vi "Channel_test_waveforms.vi"(0 "Tested channel":i32, 2 "Olfactormeter parameters":T3={"Back valve ON delays"=[0.0, 0.0, 0.0, 0.0, 0.0, 0.0, 0.0, 0.0, 0.0, 0.0, 0.0, 0.0, 0.0, 0.0, 0.0, 0.0], "Back valve OFF delays"=[0.0, 0.0, 0.0, 0.0, 0.0, 0.0, 0.0, 0.0, 0.0, 0.0, 0.0, 0.0, 0.0, 0.0, 0.0, 0.0], "Step duration (ms)"=2.0, "TTL binary step duration (ms)"=1.0, "Sampling rate (Hz)"=20000.0, "Initial delay (ms)"=250.0, "Pulse duration (ms)"=250.0} {"Initial delay (ms)" format="%#_13g"}, 3 "Odour bottles":T2(array[cluster])=[[{"Mixture components"=[{"Name"="MINERAL OIL", "CID"=0, "Volatility"=0.0}], "Name"="B1 (Bl)", "VPs"="0.0E+0", "Proportion"=[{"Numeric"=100.0}], "Selected"=FALSE, "Counter"=TRUE}, {"Mixture components"=[{"Name"="Methyl benzoate", "CID"=8103, "Volatility"=0.38}, {"Name"="Menthone", "CID"=8063, "Volatility"=0.28}], "Name"="B3 (ME2)", "VPs"="3.3E-1 ± 21%", "Proportion"=[{"Numeric"=50.0}, {"Numeric"=50.0}], "Selected"=TRUE, "Counter"=FALSE}, {"Mixture components"=[{"Name"="Decanol", "CID"=460, "Volatility"=0.00851}], "Name"="B5 (C4f)", "VPs"="8.5E-3", "Proportion"=[{"Numeric"=100.0}], "Selected"=FALSE, "Counter"=FALSE}, {"Mixture components"=[{"Name"="Acetophenone", "CID"=8174, "Volatility"=0.45}, {"Name"="Fenchone", "CID"=8635, "Volatility"=0.82}], "Name"="B7 (ME1)", "VPs"="6.4E-1 ± 41%", "Proportion"=[{"Numeric"=50.0}, {"Numeric"=50.0}], "Selected"=FALSE, "Counter"=FALSE}], [{"Mixture components"=[{"Name"="MINERAL OIL", "CID"=0, "Volatility"=0.0}], "Name"="B2 (Bl)", "VPs"="0.0E+0", "Proportion"=[{"Numeric"=100.0}], "Selected"=FALSE, "Counter"=TRUE}, {"Mixture components"=[{"Name"="Octanol", "CID"=7439, "Volatility"=0.0794}], "Name"="B4 (C4cA)", "VPs"="7.9E-2", "Proportion"=[{"Numeric"=100.0}], "Selected"=FALSE, "Counter"=FALSE}, {"Mixture components"=[{"Name"="MINERAL OIL", "CID"=0, "Volatility"=0.0}], "Name"="B6 (Bl)", "VPs"="0.0E+0", "Proportion"=[{"Numeric"=100.0}], "Selected"=FALSE, "Counter"=FALSE}, {"Mixture components"=[{"Name"="Heptanoic acid ", "CID"=957, "Volatility"=0.0107}], "Name"="B8 (C3cA)", "VPs"="1.1E-2", "Proportion"=[{"Numeric"=100.0}], "Selected"=FALSE, "Counter"=FALSE}], [{"Mixture components"=[{"Name"="MINERAL OIL", "CID"=0, "Volatility"=0.0}], "Name"="B9 (Bl)", "VPs"="0.0E+0", "Proportion"=[{"Numeric"=100.0}], "Selected"=FALSE, "Counter"=TRUE}, {"Mixture components"=[{"Name"="Geranyl acetate", "CID"=6985, "Volatility"=0.03}, {"Name"="Dimethylacetophenone", "CID"=7144, "Volatility"=0.063}], "Name"="B11 (MW1)", "VPs"="4.6E-2 ± 50%", "Proportion"=[{"Numeric"=50.0}, {"Numeric"=50.0}], "Selected"=FALSE, "Counter"=FALSE}, {"Mixture components"=[{"Name"="Geraniol", "CID"=6405, "Volatility"=0.03}, {"Name"="Phenyl butanone", "CID"=7762, "Volatility"=0.1}], "Name"="B13 (MW2)", "VPs"="6.5E-2 ± 76%", "Proportion"=[{"Numeric"=50.0}, {"Numeric"=50.0}], "Selected"=FALSE, "Counter"=FALSE}, {"Mixture components"=[{"Name"="Methylheptanoic acid", "CID"=1032, "Volatility"=0.018}], "Name"="B15 (C3f)", "VPs"="1.8E-2", "Proportion"=[{"Numeric"=100.0}], "Selected"=FALSE, "Counter"=FALSE}], [{"Mixture components"=[{"Name"="MINERAL OIL", "CID"=0, "Volatility"=0.0}], "Name"="B10 (Bl)", "VPs"="0.0E+0", "Proportion"=[{"Numeric"=100.0}], "Selected"=FALSE, "Counter"=TRUE}, {"Mixture components"=[{"Name"="Valeric acid", "CID"=8025, "Volatility"=0.196}], "Name"="B12 (C3cB)", "VPs"="2.0E-1", "Proportion"=[{"Numeric"=100.0}], "Selected"=FALSE, "Counter"=FALSE}, {"Mixture components"=[{"Name"="Nonanol", "CID"=4133, "Volatility"=0.0227}], "Name"="B14 (C4cB)", "VPs"="2.3E-2", "Proportion"=[{"Numeric"=100.0}], "Selected"=FALSE, "Counter"=FALSE}, {"Mixture components"=[{"Name"="Hydroxacetophenone", "CID"=7462, "Volatility"=0.0856}], "Name"="B16 (Ol)", "VPs"="8.6E-2", "Proportion"=[{"Numeric"=100.0}], "Selected"=FALSE, "Counter"=FALSE}]], 4 "Test type":T1(ring), 5 "Reset counters":bool) -> (7 "waveform array":digitalwaveform[](array[waveform])=[{"t0"=timestamp(0 s since 1904-01-01), "dt"=5e-05, "Y"={"transitions"=[], "data"=array5001x1[5001 elements]}, "attributes"=variant("NI_LineNames"=variant(string "Front valve 1"))}, {"t0"=timestamp(0 s since 1904-01-01), "dt"=5e-05, "Y"={"transitions"=[], "data"=array10001x1[10001 elements]}, "attributes"=variant("NI_LineNames"=variant(string "Front valve 2"))}, {"t0"=timestamp(0 s since 1904-01-01), "dt"=5e-05, "Y"={"transitions"=[], "data"=array10001x1[10001 elements]}, "attributes"=variant("NI_LineNames"=variant(string "Front valve 3"))}, {"t0"=timestamp(0 s since 1904-01-01), "dt"=5e-05, "Y"={"transitions"=[], "data"=[]}, "attributes"=variant("NI_LineNames"=variant(string "Front valve 4"))}, {"t0"=timestamp(0 s since 1904-01-01), "dt"=5e-05, "Y"={"transitions"=[], "data"=array10001x1[10001 elements]}, "attributes"=variant("NI_LineNames"=variant(string "Front valve 5"))}, {"t0"=timestamp(0 s since 1904-01-01), "dt"=5e-05, "Y"={"transitions"=[], "data"=array10001x1[10001 elements]}, "attributes"=variant("NI_LineNames"=variant(string "Front valve 6"))}, {"t0"=timestamp(0 s since 1904-01-01), "dt"=5e-05, "Y"={"transitions"=[], "data"=array10001x1[10001 elements]}, "attributes"=variant("NI_LineNames"=variant(string "Front valve 7"))}, {"t0"=timestamp(0 s since 1904-01-01), "dt"=5e-05, "Y"={"transitions"=[], "data"=array10001x1[10001 elements]}, "attributes"=variant("NI_LineNames"=variant(string "Front valve 8"))}, {"t0"=timestamp(0 s since 1904-01-01), "dt"=5e-05, "Y"={"transitions"=[], "data"=array10001x1[10001 elements]}, "attributes"=variant("NI_LineNames"=variant(string "Front valve 9"))}, {"t0"=timestamp(0 s since 1904-01-01), "dt"=5e-05, "Y"={"transitions"=[], "data"=array10001x1[10001 elements]}, "attributes"=variant("NI_LineNames"=variant(string "Front valve 10"))}, {"t0"=timestamp(0 s since 1904-01-01), "dt"=5e-05, "Y"={"transitions"=[], "data"=array10001x1[10001 elements]}, "attributes"=variant("NI_LineNames"=variant(string "Front valve 11"))}, {"t0"=timestamp(0 s since 1904-01-01), "dt"=5e-05, "Y"={"transitions"=[], "data"=array10001x1[10001 elements]}, "attributes"=variant("NI_LineNames"=variant(string "Front valve 12"))}, {"t0"=timestamp(0 s since 1904-01-01), "dt"=5e-05, "Y"={"transitions"=[], "data"=array10001x1[10001 elements]}, "attributes"=variant("NI_LineNames"=variant(string "Front valve 13"))}, {"t0"=timestamp(0 s since 1904-01-01), "dt"=5e-05, "Y"={"transitions"=[], "data"=array10001x1[10001 elements]}, "attributes"=variant("NI_LineNames"=variant(string "Front valve 14"))}, {"t0"=timestamp(0 s since 1904-01-01), "dt"=5e-05, "Y"={"transitions"=[], "data"=array10001x1[10001 elements]}, "attributes"=variant("NI_LineNames"=variant(string "Front valve 15"))}, {"t0"=timestamp(0 s since 1904-01-01), "dt"=5e-05, "Y"={"transitions"=[], "data"=array10001x1[10001 elements]}, "attributes"=variant("NI_LineNames"=variant(string "Front valve 16"))}, {"t0"=timestamp(0 s since 1904-01-01), "dt"=5e-05, "Y"={"transitions"=[], "data"=[]}, "attributes"=variant("NI_LineNames"=variant(string "Back valve 1"))}, {"t0"=timestamp(0 s since 1904-01-01), "dt"=5e-05, "Y"={"transitions"=[], "data"=[]}, "attributes"=variant("NI_LineNames"=variant(string "Back valve 2"))}, {"t0"=timestamp(0 s since 1904-01-01), "dt"=5e-05, "Y"={"transitions"=[], "data"=[]}, "attributes"=variant("NI_LineNames"=variant(string "Back valve 3"))}, {"t0"=timestamp(0 s since 1904-01-01), "dt"=5e-05, "Y"={"transitions"=[], "data"=[]}, "attributes"=variant("NI_LineNames"=variant(string "Back valve 4"))}, {"t0"=timestamp(0 s since 1904-01-01), "dt"=5e-05, "Y"={"transitions"=[], "data"=[]}, "attributes"=variant("NI_LineNames"=variant(string "Back valve 5"))}, {"t0"=timestamp(0 s since 1904-01-01), "dt"=5e-05, "Y"={"transitions"=[], "data"=[]}, "attributes"=variant("NI_LineNames"=variant(string "Back valve 6"))}, {"t0"=timestamp(0 s since 1904-01-01), "dt"=5e-05, "Y"={"transitions"=[], "data"=[]}, "attributes"=variant("NI_LineNames"=variant(string "Back valve 7"))}, {"t0"=timestamp(0 s since 1904-01-01), "dt"=5e-05, "Y"={"transitions"=[], "data"=[]}, "attributes"=variant("NI_LineNames"=variant(string "Back valve 8"))}, {"t0"=timestamp(0 s since 1904-01-01), "dt"=5e-05, "Y"={"transitions"=[], "data"=[]}, "attributes"=variant("NI_LineNames"=variant(string "Back valve 9"))}, {"t0"=timestamp(0 s since 1904-01-01), "dt"=5e-05, "Y"={"transitions"=[], "data"=[]}, "attributes"=variant("NI_LineNames"=variant(string "Back valve 10"))}, {"t0"=timestamp(0 s since 1904-01-01), "dt"=5e-05, "Y"={"transitions"=[], "data"=[]}, "attributes"=variant("NI_LineNames"=variant(string "Back valve 11"))}, {"t0"=timestamp(0 s since 1904-01-01), "dt"=5e-05, "Y"={"transitions"=[], "data"=[]}, "attributes"=variant("NI_LineNames"=variant(string "Back valve 12"))}, {"t0"=timestamp(0 s since 1904-01-01), "dt"=5e-05, "Y"={"transitions"=[], "data"=[]}, "attributes"=variant("NI_LineNames"=variant(string "Back valve 13"))}, {"t0"=timestamp(0 s since 1904-01-01), "dt"=5e-05, "Y"={"transitions"=[], "data"=[]}, "attributes"=variant("NI_LineNames"=variant(string "Back valve 14"))}, {"t0"=timestamp(0 s since 1904-01-01), "dt"=5e-05, "Y"={"transitions"=[], "data"=[]}, "attributes"=variant("NI_LineNames"=variant(string "Back valve 15"))}, {"t0"=timestamp(0 s since 1904-01-01), "dt"=5e-05, "Y"={"transitions"=[], "data"=[]}, "attributes"=variant("NI_LineNames"=variant(string "Back valve 16"))}, {"t0"=timestamp(0 s since 1904-01-01), "dt"=5e-05, "Y"={"transitions"=[], "data"=[]}, "attributes"=variant("NI_LineNames"=variant(string "Odour TTL1"))}], 10 "Test name":string)   [LabVIEW 2016]
uses:
  <vilib>/Waveform/DWDTOps.llb/DWDT Append Digital Signals.vi
panel:
  out "Digital Waveform Graph":digitalwaveform(graph)={"t0"=timestamp(0 s since 1904-01-01), "dt"=5e-05, "Y"={"transitions"=array[10001 elements], "data"=array10001x15[150015 elements]}, "attributes"=variant("NI_LineNames"=variant(string "Odour TTL1,Back valve 16,Back valve 15,Back valve 14,Back valve 13,Back valve 12,Back valve 11,Back valve 10,Back valve 9,Back valve 8,Back valve 7,Back valve 6,Back valve 5,Back valve 4,Back valve 3,Back valve 2,Back valve 1,Front valve 16,Front valve 15,Front valve 14,Front valve 13,Front valve 12,Front valve 11,Front valve 10,Front valve 9,Front valve 8,Front valve 7,Front valve 6,Front valve 5,Front valve 4,Front valve 3,Front valve 2,Front valve 1"))}
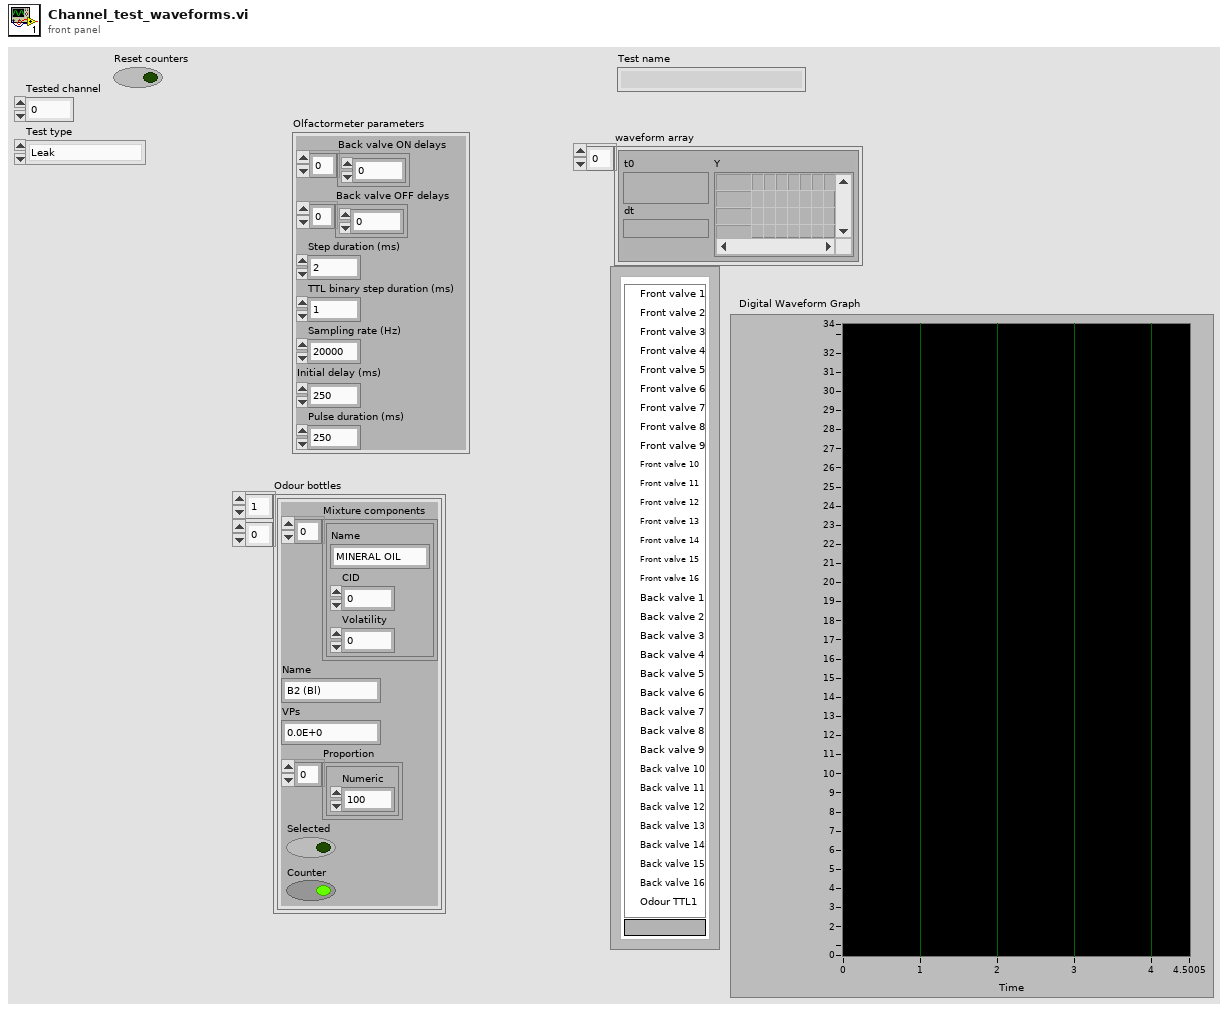
[diagram p1: front panel]
types:
  T1 = enum16{"Leak", "Flow w/o counters", "Flow w counters"}
  T2 = cluster{"Mixture components":cluster{"Name":string, "CID":i32, "Volatility":dbl}[], "Name":string, "VPs":string, "Proportion":cluster{"Numeric":dbl}[], "Selected":bool, "Counter":bool}[][]
  T3 = cluster{"Back valve ON delays":dbl[], "Back valve OFF delays":dbl[], "Step duration (ms)":dbl, "TTL binary step duration (ms)":dbl, "Sampling rate (Hz)":dbl, "Initial delay (ms)":dbl, "Pulse duration (ms)":dbl}
  T4 = cluster{"Active bottles":i32[], "Counter bottles":i32[], "All counters":i32[]}
  T5 = cluster{"Initial phase":i32, "Back-valve pre-phase ":i32, "Main phase":i32, "Back-valve post-phase":i32, "Reset":i32, "Step":i32, "Total":i32, "ON delays":i32[], "OFF delays":i32[]}
  T6 = enum16{"Inactive odour", "Active counter", "Inactive counter", "Active odour", "INVALID"}
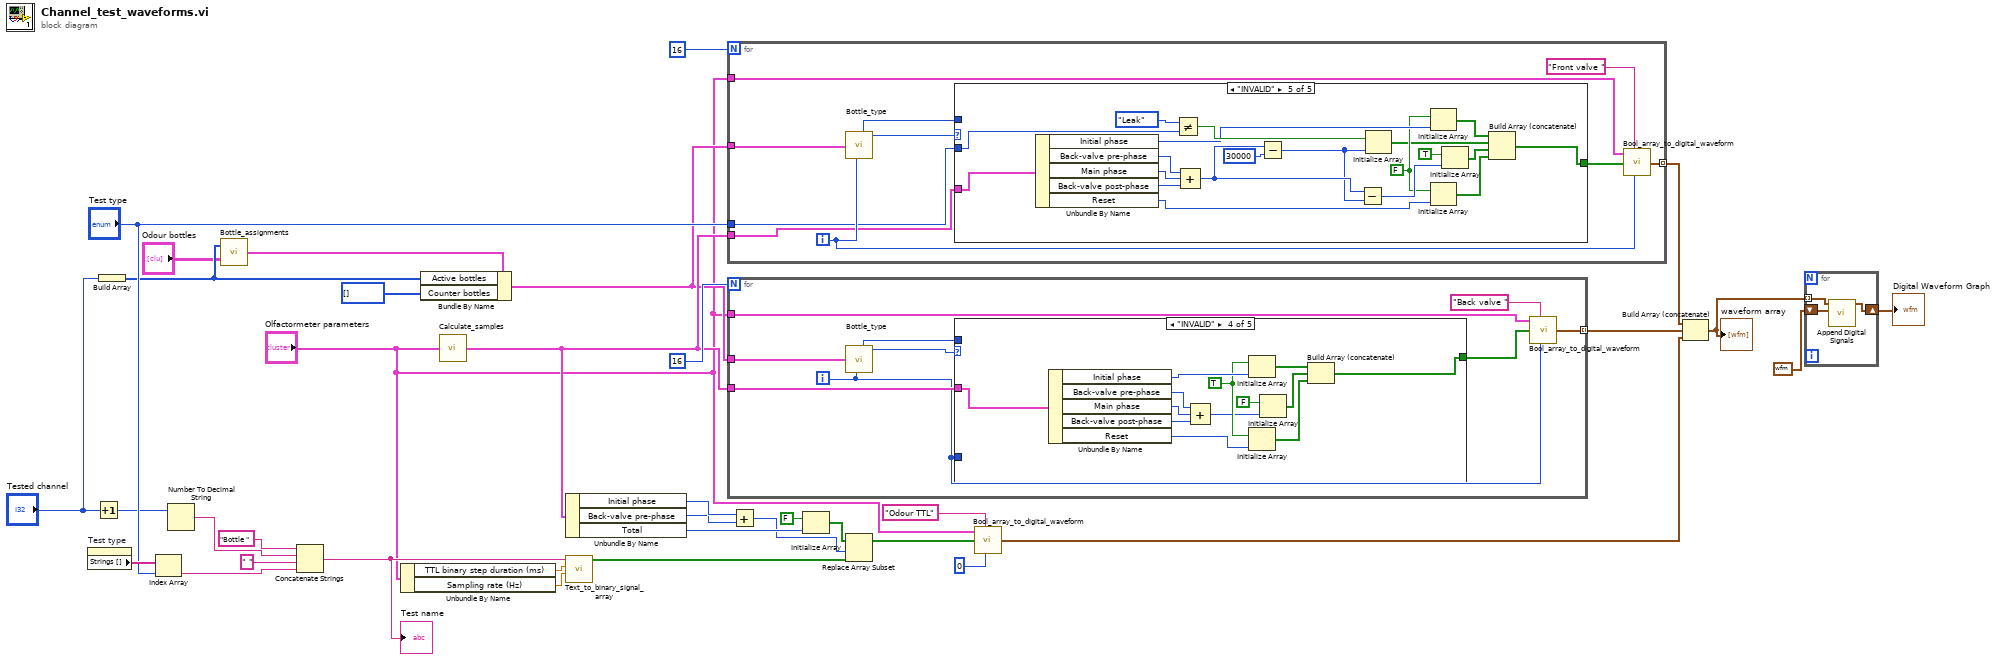
[diagram p0: block diagram]
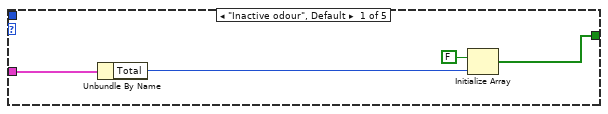
[diagram p2: hidden frame]
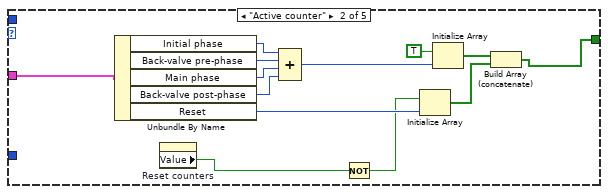
[diagram p3: hidden frame]
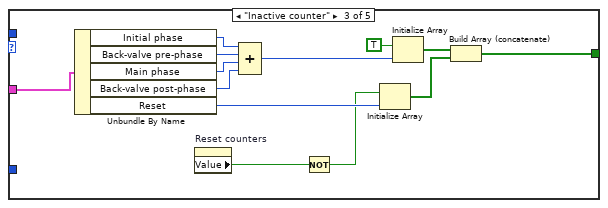
[diagram p4: hidden frame]
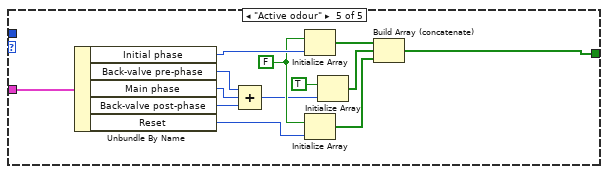
[diagram p5: hidden frame]
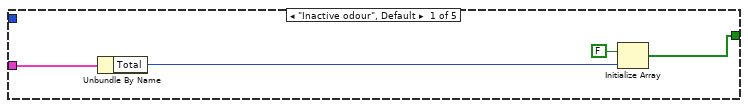
[diagram p6: hidden frame]
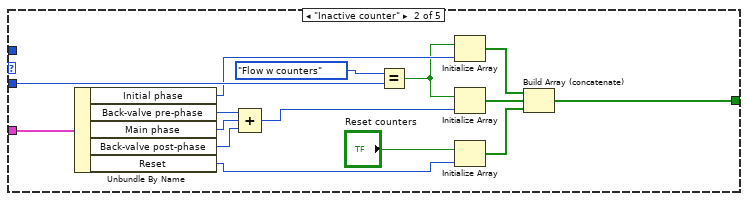
[diagram p7: hidden frame]
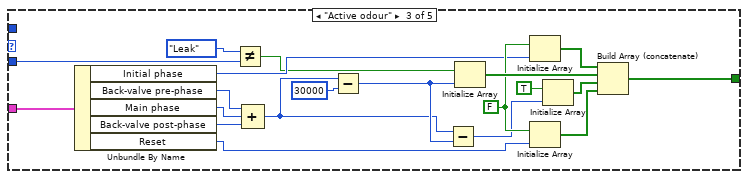
[diagram p8: hidden frame]
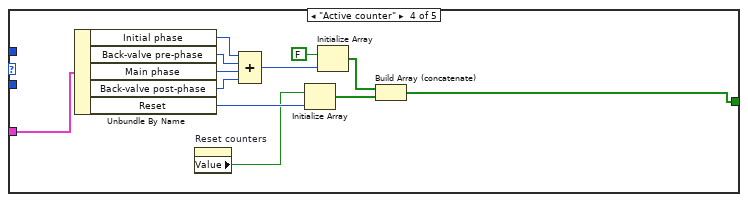
[diagram p9: hidden frame]
diagram:
  n1 = property on="Test type" class="Enum (strict)"() -> ("Strings []"=w15:string[])  [unwired: 2 in, 2 out]
  n2 = Increment(x="Tested channel") -> (x+1=w8:i32)
  n3 = Build Array("Tested channel") -> (w3:i32[])
  n4 = Index Array(array=w15, index="Test type") -> (element=w9:string)
  n5 = Number To Decimal String(number=w8) -> (decimal integer string=w11:string)  [unwired: 1 in]
  n6 = call "Bottle_assignments.vi"("Odour bottles"="Odour bottles", "Active bottles"=w3) -> ("Bottle assignments"=w1:T4)
  n7 = Concatenate Strings("Bottle " ("string"), w11, " " ("string"), w9) -> (w7:string)
  "Test name" <- w7
  n8 = Unbundle By Name("Olfactormeter parameters") -> ("TTL binary step duration (ms)"=w36:dbl, "Sampling rate (Hz)"=w33:dbl)
  n9 = Bundle By Name(cluster=w1, "Active bottles"=w3, "Counter bottles"=i32[] []) -> (w5:T4)
  n10 = call "Calculate_samples.vi"("Olfactormeter parameters"="Olfactormeter parameters") -> ("Samples"=w23:T5)  [unwired: 4 in]
  n11 = Unbundle By Name(w23) -> ("Initial phase"=w20:i32, "Back-valve pre-phase"=w19:i32, "Total"=w22:i32)
  n12 = call "Text_to_binary_signal_array.vi"("Sampling rate (Hz)"=w33, "TTL binary step duration (ms)"=w36, "Text"=w7) -> ("Signal array"=w17:bool[])  [unwired: 8 in]
  n13 = for {
    N: 16 -> [_]
    tunnel: w5 -> [w43]
    tunnel: "Olfactormeter parameters" -> [w46]
    tunnel: [w45] -> w28 mode=indexing
    tunnel: w23 -> [w40]
    tunnel: "Test type" -> [w38]
    i -> [w42]
    n14 = call "Bottle_type.vi"("Bottle assignments"=w43, "i"=w42) -> ("active bottle index"=w39:i32, "Bottle type"=w37:T6)  [unwired: 7 in]
    n15 = case shown="\"INVALID\"" w37 {
      tunnel: [w49 w56 w79 w89 w98] -> w41
      tunnel: w40 -> [w48 w57 w80 w88 w99]
      tunnel: w39 -> [_ _ _ _ _]
      tunnel: w38 -> [_ w55 w74 _ w100]
      frame "Inactive odour", Default {
        n16 = Unbundle By Name(w48) -> ("Total"=w47:i32)
        n17 = Initialize Array(FALSE, w47) -> (w49:bool[])
      }
      frame "Inactive counter" {
        n18 = Unbundle By Name(w57) -> ("Initial phase"=w52:i32, "Back-valve pre-phase"=w64:i32, "Main phase"=w63:i32, "Back-valve post-phase"=w62:i32, "Reset"=w58:i32)
        n19 = Compound Arithmetic op=ADD(w64, w63, w62) -> (w61:i32)
        n20 = Equal?(x=T1."Flow w counters", y=w55) -> (x = y?=w51:bool)
        n21 = Initialize Array(w51, w52) -> (w53:bool[])
        n22 = Initialize Array(w51, w61) -> (w60:bool[])
        n23 = Initialize Array("Reset counters", w58) -> (w59:bool[])
        n24 = Build Array (concatenate)(w53, w60, w59) -> (w56:bool[])
      }
      frame "Active odour" {
        w78 = FALSE
        n25 = Unbundle By Name(w80) -> ("Initial phase"=w77:i32, "Back-valve pre-phase"=w81:i32, "Main phase"=w82:i32, "Back-valve post-phase"=w83:i32, "Reset"=w85:i32)
        n26 = Not Equal?(x=T1."Leak", y=w74) -> (x != y?=w75:bool)
        n27 = Compound Arithmetic op=ADD(w81, w82, w83) -> (w67:i32)
        n28 = Subtract(x=w67, y=30000) -> (x-y=w68:i32)
        n29 = Subtract(x=w67, y=w68) -> (x-y=w71:i32)
        n30 = Initialize Array(w75, w68) -> (w84:bool[])
        n31 = Initialize Array(w78, w77) -> (w76:bool[])
        n32 = Initialize Array(w78, w85) -> (w70:bool[])
        n33 = Initialize Array(TRUE, w71) -> (w69:bool[])
        n34 = Build Array (concatenate)(w76, w84, w69, w70) -> (w79:bool[])
      }
      frame "Active counter" {
        n35 = Unbundle By Name(w88) -> ("Initial phase"=w97:i32, "Back-valve pre-phase"=w96:i32, "Main phase"=w95:i32, "Back-valve post-phase"=w94:i32, "Reset"=w90:i32)
        n36 = property on="Reset counters" class="Bool (strict)"() -> ("Value"=w86:bool)  [unwired: 2 in, 2 out]
        n37 = Compound Arithmetic op=ADD(w97, w96, w95, w94) -> (w93:i32)
        n38 = Initialize Array(w86, w90) -> (w91:bool[])
        n39 = Initialize Array(FALSE ("element"), w93) -> (w92:bool[])
        n40 = Build Array (concatenate)(w92, w91) -> (w89:bool[])
      }
      frame "INVALID" {
        w106 = FALSE
        n41 = Unbundle By Name(w99) -> ("Initial phase"=w107:i32, "Back-valve pre-phase"=w105:i32, "Main phase"=w104:i32, "Back-valve post-phase"=w103:i32, "Reset"=w101:i32)
        n42 = Not Equal?(x=T1."Leak", y=w100) -> (x != y?=w109:bool)
        n43 = Compound Arithmetic op=ADD(w105, w104, w103) -> (w116:i32)
        n44 = Subtract(x=w116, y=30000) -> (x-y=w115:i32)
        n45 = Subtract(x=w116, y=w115) -> (x-y=w112:i32)
        n46 = Initialize Array(w109, w115) -> (w102:bool[])
        n47 = Initialize Array(w106, w107) -> (w108:bool[])
        n48 = Initialize Array(w106, w101) -> (w113:bool[])
        n49 = Initialize Array(TRUE, w112) -> (w114:bool[])
        n50 = Build Array (concatenate)(w108, w102, w114, w113) -> (w98:bool[])
      }
    }
    n51 = call "Bool_array_to_digital_waveform.vi"("Olfactormeter parameters"=w46, "Type"="Front valve ", "odour waveform array"=w41, "i"=w42) -> ("digital waveform"=w45:digitalwaveform)  [unwired: 3 in]
  }
  n52 = for {
    N: 16 -> [_]
    tunnel: [w124] -> w32 mode=indexing
    tunnel: "Olfactormeter parameters" -> [w126]
    tunnel: w5 -> [w123]
    tunnel: w23 -> [w121]
    i -> [w119]
    n53 = call "Bottle_type.vi"("Bottle assignments"=w123, "i"=w119) -> ("active bottle index"=w122:i32, "Bottle type"=w118:T6)  [unwired: 7 in]
    n54 = case shown="\"INVALID\"" w118 {
      tunnel: w121 -> [w129 w133 w155 w158 w173]
      tunnel: w122 -> [_ _ _ _ _]
      tunnel: [w127 w132 w145 w157 w170] -> w120
      tunnel: w119 -> [_ _ _ _ _]
      frame "Inactive odour", Default {
        n55 = Unbundle By Name(w129) -> ("Total"=w128:i32)
        n56 = Initialize Array(FALSE, w128) -> (w127:bool[])
      }
      frame "Active counter" {
        n57 = Unbundle By Name(w133) -> ("Initial phase"=w142:i32, "Back-valve pre-phase"=w141:i32, "Main phase"=w140:i32, "Back-valve post-phase"=w139:i32, "Reset"=w136:i32)
        n58 = property on="Reset counters" class="Bool (strict)"() -> ("Value"=w131:bool)  [unwired: 2 in, 2 out]
        n59 = Compound Arithmetic op=ADD(w142, w141, w140, w139) -> (w138:i32)
        n60 = Not(x=w131) -> (.not. x?=w134:bool)
        n61 = Initialize Array(w134, w136) -> (w135:bool[])
        n62 = Initialize Array(TRUE, w138) -> (w137:bool[])
        n63 = Build Array (concatenate)(w137, w135) -> (w132:bool[])
      }
      frame "Inactive counter" {
        n64 = Unbundle By Name(w155) -> ("Initial phase"=w154:i32, "Back-valve pre-phase"=w153:i32, "Main phase"=w152:i32, "Back-valve post-phase"=w151:i32, "Reset"=w148:i32)
        n65 = property on="Reset counters" class="Bool (strict)"() -> ("Value"=w147:bool)  [unwired: 2 in, 2 out]
        n66 = Compound Arithmetic op=ADD(w154, w153, w152, w151) -> (w150:i32)
        n67 = Not(x=w147) -> (.not. x?=w144:bool)
        n68 = Initialize Array(w144, w148) -> (w146:bool[])
        n69 = Initialize Array(TRUE, w150) -> (w149:bool[])
        n70 = Build Array (concatenate)(w149, w146) -> (w145:bool[])
      }
      frame "INVALID" {
        w167 = TRUE
        n71 = Unbundle By Name(w158) -> ("Initial phase"=w168:i32, "Back-valve pre-phase"=w166:i32, "Main phase"=w165:i32, "Back-valve post-phase"=w164:i32, "Reset"=w161:i32)
        n72 = Compound Arithmetic op=ADD(w166, w165, w164) -> (w163:i32)
        n73 = Initialize Array(w167, w168) -> (w169:bool[])
        n74 = Initialize Array(w167, w161) -> (w162:bool[])
        n75 = Initialize Array(FALSE ("element"), w163) -> (w159:bool[])
        n76 = Build Array (concatenate)(w169, w159, w162) -> (w157:bool[])
      }
      frame "Active odour" {
        w180 = FALSE
        n77 = Unbundle By Name(w173) -> ("Initial phase"=w181:i32, "Back-valve pre-phase"=w179:i32, "Main phase"=w178:i32, "Back-valve post-phase"=w177:i32, "Reset"=w174:i32)
        n78 = Compound Arithmetic op=ADD(w179, w178, w177) -> (w176:i32)
        n79 = Initialize Array(w180, w181) -> (w182:bool[])
        n80 = Initialize Array(w180, w174) -> (w175:bool[])
        n81 = Initialize Array(TRUE ("element"), w176) -> (w171:bool[])
        n82 = Build Array (concatenate)(w182, w171, w175) -> (w170:bool[])
      }
    }
    n83 = call "Bool_array_to_digital_waveform.vi"("Olfactormeter parameters"=w126, "Type"="Back valve ", "odour waveform array"=w120, "i"=w119) -> ("digital waveform"=w124:digitalwaveform)  [unwired: 3 in]
  }
  n84 = Add(x=w20, y=w19) -> (x+y=w18:i32)
  n85 = Initialize Array(FALSE, w22) -> (w21:bool[])
  n86 = Replace Array Subset(array=w21, new element=w17, index=w18) -> (w16:bool[])
  n87 = call "Bool_array_to_digital_waveform.vi"("Olfactormeter parameters"="Olfactormeter parameters", "Type"="Odour TTL" ("name"), "odour waveform array"=w16, "i"=0) -> ("digital waveform"=w25:digitalwaveform)  [unwired: 3 in]
  n88 = Build Array (concatenate)(w28, w32, w25) -> (w30:digitalwaveform[])
  "waveform array" <- w30
  n89 = for {
    shift-right: [w185] -> w29
    shift-left: digitalwaveform {"t0"=timestamp(0 s since 1904-01-01), "dt"=0.0, "Y"={"transitions"=[], "data"=[]}} ("waveform out") -> [w184]
    tunnel: w30 -> [w183] mode=indexing
    n90 = call-poly <vilib>:"Append Digital Signals.vi"("digital waveform (low bits)"=w184, "digital waveform (high bits)"=w183) -> ("digital waveform out"=w185:digitalwaveform)  [unwired: 8 in, 1 out]
  }
  "Digital Waveform Graph" <- w29
